vi "Set Image.vi"(8 "error in (no error)":errorcluster, 11 "CCDCamera in":refnum<class "Ixon_Ultra.lvclass">) -> (0 "error out":errorcluster, 3 "CCDCamera out":refnum<class "Ixon_Ultra.lvclass">)   [LabVIEW 2018, in "Ixon_Ultra.lvclass"]
doc: "Set the dimensions of the image\n\nWith this function, it is possible to set the inital column, inital line, final column and final line. Also, the vertical and horizontal binning of the pixels can be set."
uses:
  Ixon_Ultra.lvclass
  C:/Users/Denis/Desktop/S4ACS/S4ACS/Simulated_CCD_Camera/Simulated Camera.lvclass
  Simulated_CCD_Camera/Simulated Camera.lvclass
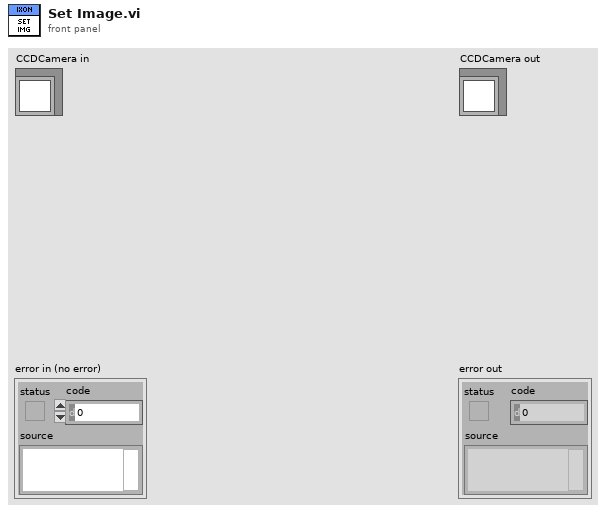
[diagram p1: front panel]
types:
  T1 = cluster{"PREAMP":u16, "READOUT_RATE":u16, "VERTICAL_SHIFT_SPEED":u16, "READ_MODE":u16, "VERTICAL_CLOCK_VOLTAGE":u16, "ACQUISITION_MODE":u16, "AD_CHANNEL":u16, "SHUTTER_TTL":u16, "SHUTTER_OPENING_TIME":u16, "SHUTTER_CLOSING_TIME":u16, "SHUTTER_MODE":u16, "TRIGGER_MODE":u16, "VBIN":u16, "INITIAL_LINE":u16, "INITIAL_COLUMN":u16, "FINAL_LINE":u16, "FINAL_COLUMN":u16, "HBIN":u16, "TEMP":u16, "COOLER_POWER_STATUS":u16}
  T2 = cluster{"PREAMP":u16, "READOUT_RATE":u16, "EM_GAIN":u16, "VERTICAL_SHIFT_SPEED":u16, "READ_MODE":u16, "FRAME_TRANSFER":bool, "VERTICAL_CLOCK_VOLTAGE":u16, "ACQUISITION_MODE":u16, "AD_CHANNEL":u16, "EM_MODE":u16, "SHUTTER_TTL":u16, "SHUTTER_OPENING_TIME":u16, "SHUTTER_CLOSING_TIME":u16, "SHUTTER_MODE":u16, "TRIGGER_MODE":u16, "VBIN":u16, "INITIAL_LINE":u16, "INITIAL_COLUMN":u16, "FINAL_LINE":u16, "FINAL_COLUMN":u16, "HBIN":u16}
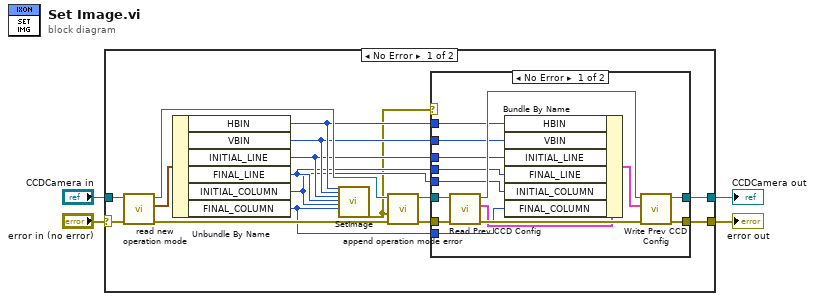
[diagram p0: block diagram]
diagram:
  n1 = case shown="No Error" "error in (no error)" {
    selector: "error in (no error)" -> [w19 w38]
    tunnel: [w12 w38] -> w4
    tunnel: "CCDCamera in" -> [w20 w37]
    tunnel: [w13 w37] -> w3
    frame No Error {
      n2 = call "read new operation mode.vi"("error in (no error)"=w19, "CCDCamera in"=w20) -> ("error out"=w16:errorcluster, "new operation mode"=w18:T1, "CCDCamera out"=w17:refnum<class "Ixon_Ultra.lvclass">)  [unwired: 7 in]
      n3 = Unbundle By Name(w18) -> ("HBIN"=w11:u16, "VBIN"=w10:u16, "INITIAL_LINE"=w9:u16, "FINAL_LINE"=w8:u16, "INITIAL_COLUMN"=w7:u16, "FINAL_COLUMN"=w6:u16)
      n4 = call <userlib>:"SetImage.vi"("hbin"=w11, "vbin"=w10, "hstart"=w9, "hend"=w8, "vstart"=w7, "vend"=w6) -> ("error out"=w5:errorcluster)  [unwired: 20 in, 1 out]
      n5 = call "append operation mode error.vi"("error in (no error)"=w16, "error"=w5, "Simulated_CCD_Camera in"=w17) -> ("error out"=w14:errorcluster, "Simulated_CCD_Camera out"=w15:refnum<class "Ixon_Ultra.lvclass">)  [unwired: 7 in]
      n6 = case shown="No Error" w5 {
        tunnel: w15 -> [w34 w36]
        tunnel: w14 -> [w33 w35]
        tunnel: [w31 w36] -> w13
        tunnel: [w29 w35] -> w12
        tunnel: w11 -> [w26 _]
        tunnel: w10 -> [w25 _]
        tunnel: w9 -> [w24 _]
        tunnel: w8 -> [w23 _]
        tunnel: w7 -> [w22 _]
        tunnel: w6 -> [w21 _]
        frame No Error {
          n7 = call-dynamic "Read Prev CCD Config.vi"("error in (no error)"=w33, "Simulated_CCD_Camera in"=w34) -> ("error out"=w30:errorcluster, "Prev CCD Config"=w28:T2, "Simulated_CCD_Camera out"=w32:refnum<class "Ixon_Ultra.lvclass">)  [unwired: 7 in]
          n8 = Bundle By Name(cluster=w28, "HBIN"=w26, "VBIN"=w25, "INITIAL_LINE"=w24, "FINAL_LINE"=w23, "INITIAL_COLUMN"=w22, "FINAL_COLUMN"=w21) -> (w27:T2)
          n9 = call-dynamic "Write Prev CCD Config.vi"("error in (no error)"=w30, "Prev CCD Config"=w27, "Simulated_CCD_Camera in"=w32) -> ("error out"=w29:errorcluster, "Simulated_CCD_Camera out"=w31:refnum<class "Ixon_Ultra.lvclass">)  [unwired: 7 in]
        }
        frame Error {
        }
      }
    }
    frame Error {
    }
  }
  "error out" <- w4
  "CCDCamera out" <- w3
